vi "Init Data Object.vi"(11 "PAS Data in":refnum<class "PAS Data.lvclass">=refnum) -> (3 "PAS Data out":refnum<class "PAS Data.lvclass">)   [LabVIEW 2014, in "PAS Data.lvclass"]
uses:
  PAS Data.lvclass
  Data/Data.lvclass
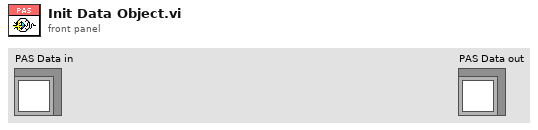
[diagram p1: front panel]
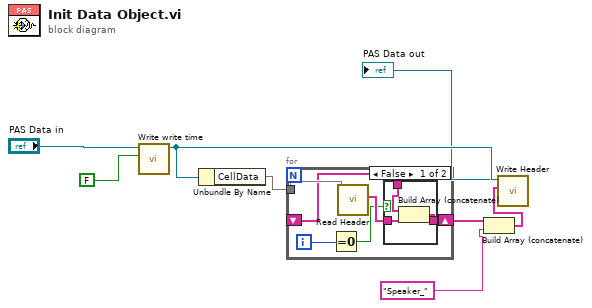
[diagram p0: block diagram]
diagram:
  n1 = call "Write write time.vi"("write time"=FALSE, "Data in"="PAS Data in") -> ("Data out"=w2:refnum<class "Data.lvclass">)  [unwired: 8 in, 1 out]
  n2 = Unbundle By Name(w2) -> ("CellData"=w6)
  n3 = for {
    tunnel: w6 -> [w14]
    shift-right: [w10] -> w5
    shift-left: _ -> [w9]
    i -> [w13]
    n4 = Equal To 0?(x=w13) -> (x = 0?=w11:bool)
    n5 = call "Read Header.vi"("Data in"=w14) -> ("Header"=w12:string[])  [unwired: 8 in, 2 out]
    n6 = case shown="False" w11 {
      tunnel: w12 -> [w15 w18]
      tunnel: [w16 w18] -> w10
      tunnel: w9 -> [w17 _]
      frame False {
        n7 = Build Array (concatenate)(w17, w15) -> (w16:string[])
      }
      frame True {
      }
    }
  }
  n8 = Build Array (concatenate)(w5, "Speaker_") -> (w3:string[])
  n9 = call "Write Header.vi"("Header"=w3, "Data in"=w2) -> ("Data out"=→"PAS Data out":refnum<class "Data.lvclass">)  [unwired: 8 in, 1 out]
